vi "Multi_Histogram.vi"(6 "Equi Spaced":dbl[][](array[numeric]) format="%.2f", 7 "Vari Spaced":dbl[][](array[numeric]) format="%.2f") -> (3 "Histogram":dbl[][](array[numeric]) format="%.2f")   [LabVIEW 2010]
uses:
  Globals/Meas_global.vi
  <vilib>/Analysis/NI_AALBase.lvlib
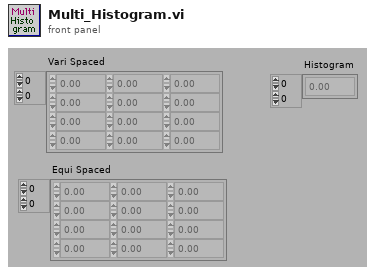
[diagram p1: front panel]
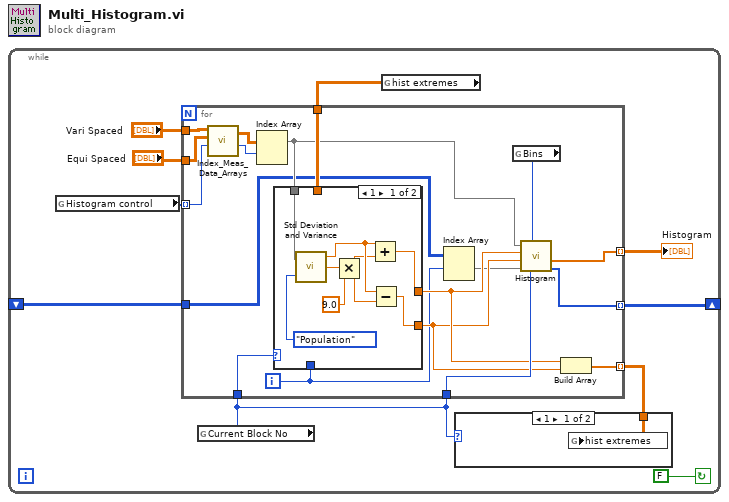
[diagram p0: block diagram]
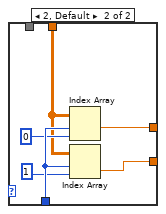
[diagram p3: hidden frame]
diagram:
  n1 = while {
    shift-left: _ -> [w5]
    shift-right: [w9] -> _
    stop <- FALSE continue-if-true
    n2 = global read "Meas_global.vi" "Histogram control"() -> (w7:i32[])
    n3 = global read "Meas_global.vi" "Current Block No"() -> (w2:i32)
    n4 = global read "Meas_global.vi" "hist extremes"() -> (w6:dbl[][])
    n5 = for {
      tunnel: w7 -> [w13] mode=indexing
      tunnel: [w17] -> w10 mode=indexing
      tunnel: w2 -> [w29]
      tunnel: [w28] -> w9 mode=indexing
      tunnel: w2 -> [w27]
      tunnel: [w24] -> w8 mode=indexing
      tunnel: w6 -> [w23]
      tunnel: w5 -> [w20]
      tunnel: "Vari Spaced" -> [w15]
      tunnel: "Equi Spaced" -> [w14]
      i -> [w19]
      n6 = call "Index_Meas_Data_Arrays.vi"("1st Desired Index"=w13, "Equi Spaced"=w14, "Vari Spaced"=w15) -> ("1st Output Index"=w12:i32, "Output Array"=w16:dbl[][])  [unwired: 1 in, 2 out]
      n7 = Index Array(array=w16, index (row)=w12) -> (element=w21:dbl[])  [unwired: 1 in]
      n8 = case shown="1" w27 {
        tunnel: [w32 w43] -> w26
        tunnel: [w31 w42] -> w25
        tunnel: w19 -> [_ w41]
        tunnel: w21 -> [w37 _]
        tunnel: w23 -> [_ w38]
        frame 1 {
          n9 = call <vilib>:"Std Deviation and Variance.vi"("X"=w37, "Weighting (Sample)"=enum16{"Sample", "Population"}."Population") -> ("mean"=w36:dbl, "standard deviation"=w35:dbl)  [unwired: 1 out]
          n10 = Multiply(x=w35, y=9.0) -> (x*y=w33:dbl)
          n11 = Add(x=w36, y=w33) -> (x+y=w32:dbl)
          n12 = Subtract(x=w36, y=w33) -> (x-y=w31:dbl)
        }
        frame 2, Default {
          n13 = Index Array(array=w38, index (row)=w41, index (col)=0) -> (element=w43:dbl)
          n14 = Index Array(array=w38, index (row)=w41, index (col)=1) -> (element=w42:dbl)
        }
      }
      n15 = Index Array(array=w20, index (row)=w19) -> (element=w18:i32[])  [unwired: 1 in]
      n16 = global read "Meas_global.vi" "Bins"() -> (w22:i32)
      n17 = call "Histogram.vi"("Current Block No"=w29, "No of bins"=w22, "Shift Hist"=w18, "Min value"=w25, "Max value"=w26, "X"=w21) -> ("Shift Hist"=w28:i32[], "Histogram of X"=w17:dbl[])  [unwired: 1 in, 2 out]
      n18 = Build Array(w26, w25) -> (w24:dbl[])
    }
    "Histogram" <- w10
    n19 = case shown="1" w2 {
      tunnel: w8 -> [w11 _]
      frame 1 {
        n20 = global write "Meas_global.vi" "hist extremes"(w11) -> ()
      }
      frame 2, Default {
      }
    }
  }
